vi "Get Initialized.vi"(8 "error in":errorcluster, 11 "Simulated CANopen Node in":refnum<class "Simulated CANopen Node.lvclass">) -> (0 "error out":errorcluster, 2 "Initialized":bool, 3 "Simulated CANopen Node out":refnum<class "Simulated CANopen Node.lvclass">)   [LabVIEW 2020, in "Simulated CANopen Node.lvclass"]
uses:
  Simulated CANopen Node.lvclass
  Simulated CANopen Node.lvclass/Simulated CANopen Node.ctl
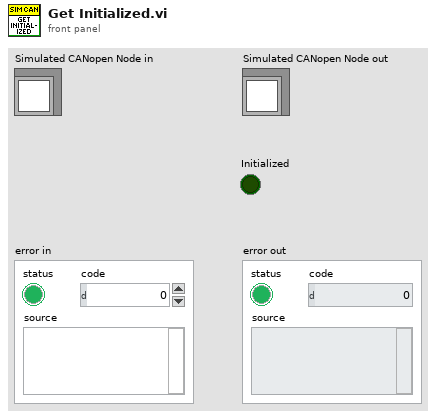
[diagram p1: front panel]
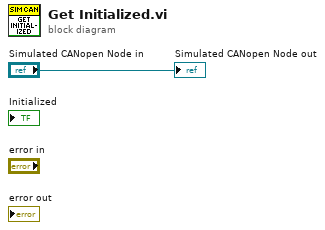
[diagram p0: block diagram]
diagram:
  "Simulated CANopen Node out" <- "Simulated CANopen Node in"
